vi "Global_Status.vi"() -> ()   [LabVIEW 2012]
panel:
  out "Motor ON":bool
  out "CCD_ON":bool
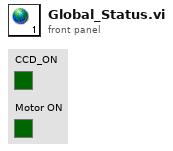
[diagram p1: front panel]
diagram:
